vi "Drive Off HAB2.vi"(6 "Right Current Drawn":dbl=7.625, 7 "Left Position":dbl=-148.0, 8 "Right Velocity":dbl, 9 "Right Position":dbl=-81.0, 10 "Left Current Drawn":dbl=5.125, 11 "Left Velocity":dbl) -> (0 "Right Output":dbl=-0.3, 1 "Zero Encoders":bool=TRUE, 2 "Control Mode":T1=15 items=["PercentOutput"=0, "Position"=1, "Velocity"=2, "Current"=3, "Follower"=5, "MotionProfile"=6, "MotionMagic"=7, "MotionProfileArc"=10, "Disabled"=15], 3 "Left Output":dbl=-0.3, 4 "DONE":bool=TRUE, 5 "Step":enum16{"Go Forward", "Go Backward", "Set Home"}(ring)=enum."Go Backward")   [LabVIEW 2018]
uses:
  <vilib>/Rock Robotics/WPI/ThirdParty/Phoenix-LabVIEW/Motor Controller/Controls/CTRE_Phoenix_MotorControl_ControlMode.ctl
panel:
  in  "Time to wait before thinking I stopped ms":u32=250
  in  "Moving Backwards throttle":dbl=-0.35
  in  "Right MM Setpoint":dbl=8100.0
  in  "Left MM Setpoint":dbl=8100.0
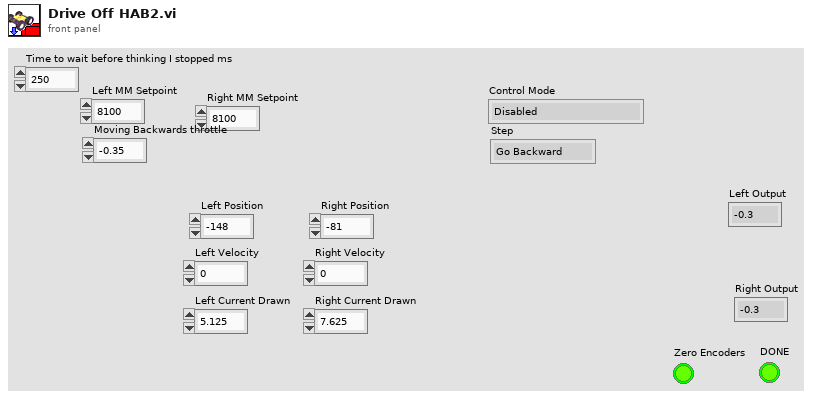
[diagram p1: front panel]
types:
  T1 = typedef "CTRE_Phoenix_MotorControl_ControlMode.ctl" = u16
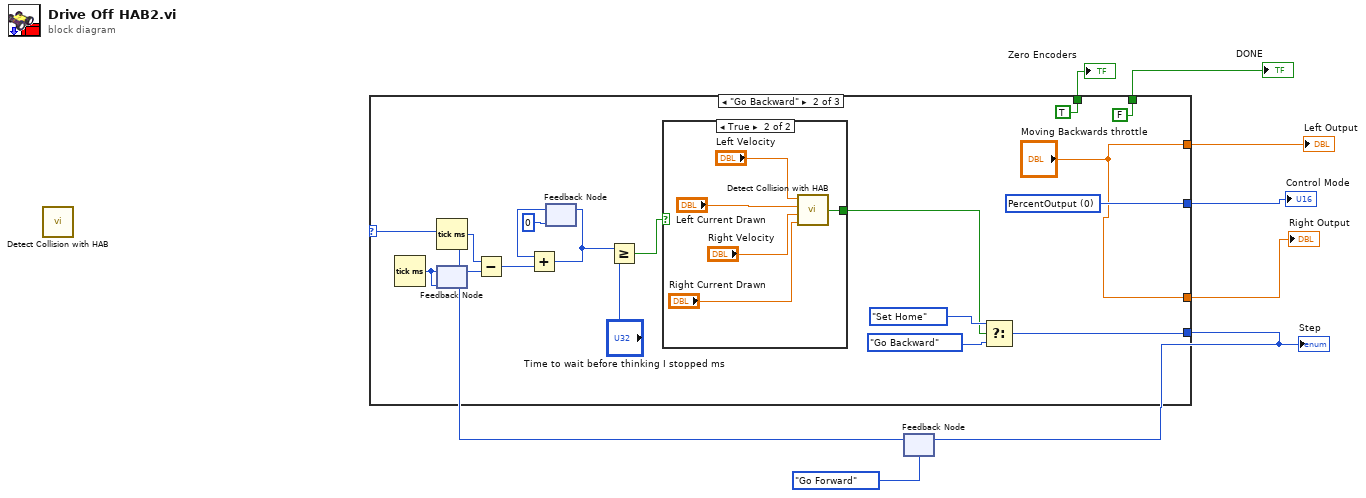
[diagram p0: block diagram]
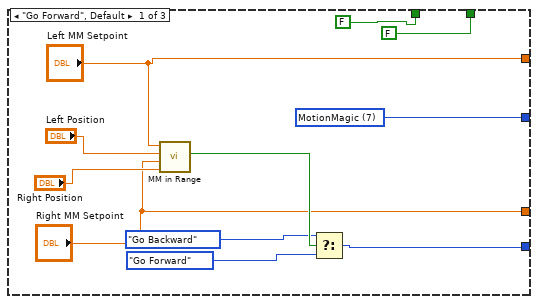
[diagram p2: hidden frame]
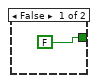
[diagram p3: hidden frame]
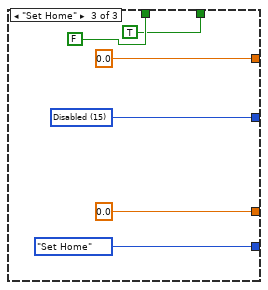
[diagram p4: hidden frame]
diagram:
  n1 = call "Detect Collision with HAB.vi"() -> ()  [unwired: 4 in, 1 out]
  n2 = feedback #1(enum16{"Go Forward", "Go Backward", "Set Home"}."Go Forward") -> (w5:enum16{"Go Forward", "Go Backward", "Set Home"})
  n3 = case shown="\"Go Backward\"" w5 {
    tunnel: [w19 w36 w47] -> w8
    tunnel: ["Left MM Setpoint" "Moving Backwards throttle" 0.0 ("Left Output")] -> w7
    tunnel: ["Right MM Setpoint" "Moving Backwards throttle" 0.0 ("Right Output")] -> w6
    tunnel: [w15 w35 enum16{"Go Forward", "Go Backward", "Set Home"}."Set Home"] -> w4
    tunnel: [FALSE ("DONE/Zero Encoders") TRUE ("DONE/Zero Encoders") FALSE ("DONE/Zero Encoders")] -> w2
    tunnel: [FALSE ("DONE/Zero Encoders") FALSE ("DONE/Zero Encoders") TRUE ("DONE/Zero Encoders")] -> w1
    frame "Go Forward", Default {
      w19 = T1 7 items=["PercentOutput"=0, "Position"=1, "Velocity"=2, "Current"=3, "Follower"=5, "MotionProfile"=6, "MotionMagic"=7, "MotionProfileArc"=10, "Disabled"=15] ("Control Mode")
      n4 = call "MM in Range.vi"("Right Position"="Right Position", "Right Setpoint"="Right MM Setpoint", "Left position"="Left Position", "Left Setpoint"="Left MM Setpoint") -> ("\"Done with step\" enough"=w18:bool)  [unwired: 7 in]
      n5 = Select(t=enum16{"Go Forward", "Go Backward", "Set Home"}."Go Backward", s=w18, f=enum16{"Go Forward", "Go Backward", "Set Home"}."Go Forward") -> (s? t:f=w15:enum16{"Go Forward", "Go Backward", "Set Home"})
    }
    frame "Go Backward" {
      w36 = T1 0 items=["PercentOutput"=0, "Position"=1, "Velocity"=2, "Current"=3, "Follower"=5, "MotionProfile"=6, "MotionMagic"=7, "MotionProfileArc"=10, "Disabled"=15] ("Control Mode")
      n6 = Tick Count (ms)() -> (millisecond timer value=w23:u32)
      n7 = Tick Count (ms)() -> (millisecond timer value=w27:u32)
      n8 = feedback-in #2(w23) -> ()
      n9 = feedback #2(w23) -> (w28:u32)
      n10 = Subtract(x=w27, y=w28) -> (x-y=w26:u32)
      n11 = feedback #3(u32 0) -> (w25:u32)
      n12 = Add(x=w25, y=w26) -> (x+y=w21:u32)
      n13 = feedback-in #3(w21) -> ()
      n14 = Greater Or Equal?(x=w21, y="Time to wait before thinking I stopped ms") -> (x >= y?=w22:bool)
      n15 = case shown="True" w22 {
        tunnel: [FALSE w42] -> w32
        frame False {
        }
        frame True {
          n16 = call "Detect Collision with HAB.vi"("Right Current"="Right Current Drawn", "Right Velocity"="Right Velocity", "Left Current"="Left Current Drawn", "Left Velocity"="Left Velocity") -> ("HIT WALL"=w42:bool)
        }
      }
      n17 = Select(t=enum16{"Go Forward", "Go Backward", "Set Home"}."Set Home", s=w32, f=enum16{"Go Forward", "Go Backward", "Set Home"}."Go Backward") -> (s? t:f=w35:enum16{"Go Forward", "Go Backward", "Set Home"})
    }
    frame "Set Home" {
      w47 = T1 15 items=["PercentOutput"=0, "Position"=1, "Velocity"=2, "Current"=3, "Follower"=5, "MotionProfile"=6, "MotionMagic"=7, "MotionProfileArc"=10, "Disabled"=15] ("Control Mode")
    }
  }
  "Left Output" <- w7
  "Right Output" <- w6
  "Control Mode" <- w8
  "Zero Encoders" <- w2
  "Step" <- w4
  "DONE" <- w1
  n18 = feedback-in #1(w4) -> ()
